vi "IMU Parsing.vi"() -> (0 "IMU error out":errorcluster)   [LabVIEW 2016]
uses:
  <vilib>/Platform/TimedLoop/XDataNode/timing_clust.ctl
  <vilib>/Platform/TimedLoop/XDataNode/nitl_modes.ctl
  <vilib>/Platform/TimedLoop/XDataNode/wakeup.ctl
  <vilib>/Platform/TimedLoop/XDataNode/XDataNode.xnode
  <vilib>/Platform/TimedLoop/XDataNode/XDNodeRunTimeDep.lvlib
panel:
  in  "stop?":bool
  in  "IMU error in":errorcluster
  in  "IMU Baud rate":u32(ring)=9600 items=["Auto Connect"=0, "300"=300, "600"=600, "1200"=1200, "2400"=2400, "4800"=4800, "9600"=9600, "19200"=19200, "38400"=38400, "57600"=57600, "115200"=115200]
  out "IMU port out":refnum<visa-resource-name>
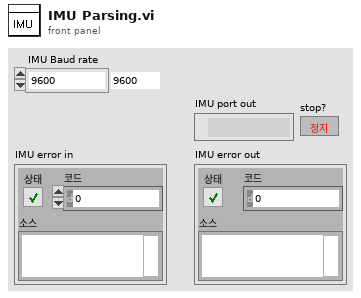
[diagram p1: front panel]
types:
  T1 = typedef "XDNodeRunTimeDep.lvlib/timing_clust.ctl" = cluster{"Expected End [f-1]":u64, "Actual End [f-1]":u64, "Finished Late? [f-1]":bool, "Expected End [i-1]":u64, "Actual End [i-1]":u64, "Finished Late? [i-1]":bool, "Expected Start [i]":u64, "Actual Start [i]":u64, "Expected Start [f]":u64, "Actual Start [f]":u64, "Source Name":string, "Structure Name":string, "Period":i64, "Deadline":i64, "Offset":i64, "Start":i64, "Priority":i32, "Timeout":i32, "Mode":T2, "Wakeup Reason":T3, "Error":errorcluster, "Source Type":string, "Secondary Source Type":string, "Global End Time":u64, "Global Start Time":u64, "Frame Duration":u64, "Iteration Duration":u64, "Assigned CPU":i32, "I/O Scan Engine Mode":u32}
  T2 = typedef "XDNodeRunTimeDep.lvlib/nitl_modes.ctl" = enum32{"No Change", "Process missed periods, maintain original phase", "Discard missed periods, maintain original phase", "Process missed periods, ignore original phase", "Discard missed periods, ignore original phase"}
  T3 = typedef "XDNodeRunTimeDep.lvlib/wakeup.ctl" = enum32{"Normal", "Aborted", "Asynchronous wakeup", "Timing source error", "Timed loop error", "Timeout"}
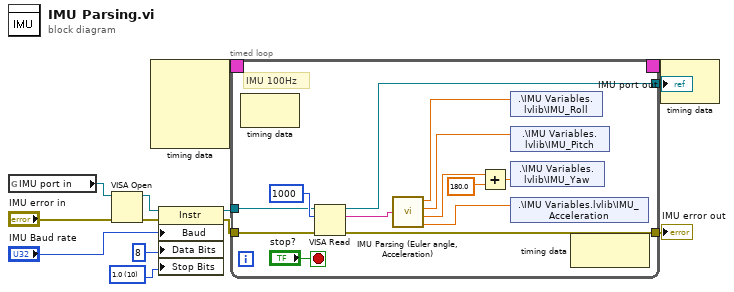
[diagram p0: block diagram]
diagram:
  w11 = u16 10 items=["1.0"=10, "1.5"=15, "2.0"=20] ("Serial Settings:Stop Bits")
  n1 = global read "[GV]_IMU Port NUM.vi" "IMU port in"() -> (w3:refnum<visa-resource-name>)
  n2 = VISA Open(error in (no error)="IMU error in", VISA resource name=w3) -> (VISA resource name=w10:refnum<visa-resource-name>, error out=w8:errorcluster)  [unwired: 3 in]
  n3 = node-c288() -> (w2:T1)  [unwired: 4 in]
  n4 = property class="Instr"(reference=w10, error in=w8, "Baud"="IMU Baud rate", "Data Bits"=u16 8 ("Serial Settings:Data Bits"), "Stop Bits"=w11) -> (reference out=w6:refnum<visa-resource-name>, error out=w5:errorcluster)
  n5 = timed-loop {
    tunnel: w6 -> [w25]
    tunnel: w5 -> [w24]
    tunnel: [w23] -> w4
    tunnel: [w22] -> w13
    timing: w2 -> [_]
    timing-out: [_] -> w1
    stop <- "stop?" stop-if-true
    # "IMU 100Hz"
    n6 = node-c288() -> ()  [unwired: 1 in, 1 out]
    n7 = VISA Read(VISA resource name=w25, byte count=u32 1000 ("바이트 카운트"), error in (no error)=w24) -> (VISA resource name out=w22:refnum<visa-resource-name>, read buffer=w21:string, error out=w23:errorcluster)  [unwired: 1 out]
    n8 = call "IMU Parsing (Euler angle, Acceleration).vi"("IMU Data"=w21) -> ("IMU_Roll"=w16:dbl, "IMU_Pitch"=w18:dbl, "IMU_Yaw"=w19:dbl, "IMU Raw ax"=w15:dbl)  [unwired: 4 in]
    n9 = Add(x=w19, y=180.0) -> (x+y=w17:dbl)
    n10 = shared-variable ".\\IMU Variables.lvlib\\IMU_Roll"(w16) -> ()  [unwired: 1 in, 1 out]
    n11 = shared-variable ".\\IMU Variables.lvlib\\IMU_Pitch"(w18) -> ()  [unwired: 1 in, 1 out]
    n12 = shared-variable ".\\IMU Variables.lvlib\\IMU_Yaw"(w17) -> ()  [unwired: 1 in, 1 out]
    n13 = shared-variable ".\\IMU Variables.lvlib\\IMU_Acceleration"(w15) -> ()  [unwired: 1 in, 1 out]
    n14 = node-c288() -> ()  [unwired: 1 in, 1 out]
  }
  "IMU port out" <- w13
  "IMU error out" <- w4
  n15 = node-c288(w1) -> ()  [unwired: 1 out]
